vi "Build Param Properties.vi"(0 "Parameter":T1, 5 "error in (no error)":errorcluster) -> (7 "signed":bool, 8 "Prop Names":string[](array[string]), 9 "numberBits":i32, 10 "Prop Values":variant[](array[variant]), 11 "startBit":i32, 13 "scaleFactor":dbl, 16 "name":string, 18 "error out":errorcluster, 19 "scaleOffset":dbl)   [LabVIEW 2013, in "AIT 664 Custom Device.lvlib"]
uses:
  AIT 664 Custom Device.lvlib
  Controls/664 -Param.ctl
  Controls and Global/Global.vi
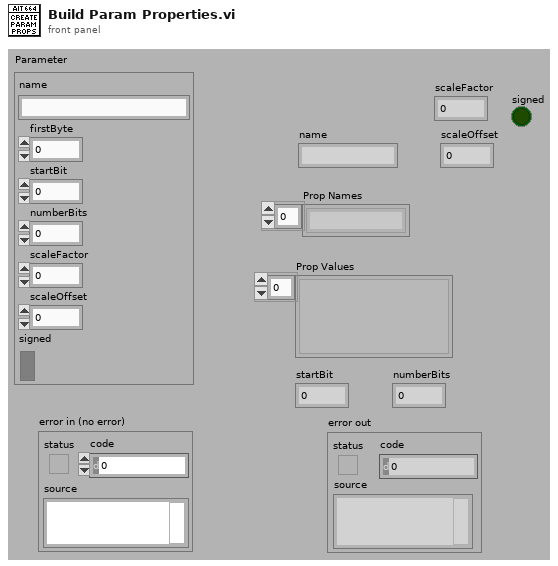
[diagram p1: front panel]
types:
  T1 = typedef "AIT 664 Custom Device.lvlib/664 -Param.ctl" = cluster{"name":string, "firstByte":i32, "startBit":i32, "numberBits":i32, "scaleFactor":dbl, "scaleOffset":dbl, "signed":bool}
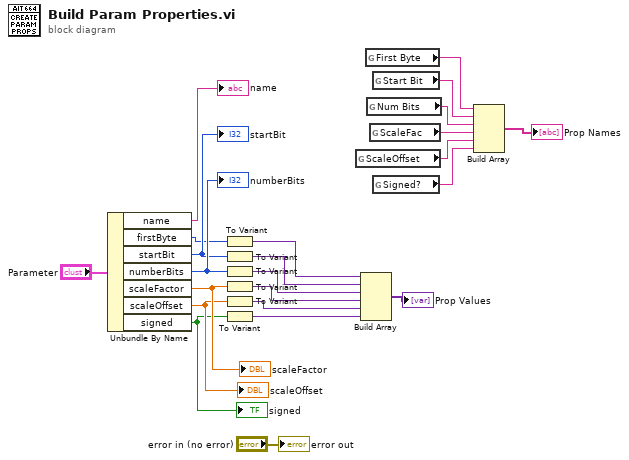
[diagram p0: block diagram]
diagram:
  n1 = Unbundle By Name("Parameter") -> ("name"=→"name":string, "firstByte"=w2:i32, "startBit"=w18:i32, "numberBits"=w22:i32, "scaleFactor"=w12:dbl, "scaleOffset"=w11:dbl, "signed"=w7:bool)
  "startBit" <- w18
  "numberBits" <- w22
  "scaleOffset" <- w11
  "scaleFactor" <- w12
  "signed" <- w7
  n2 = To Variant(anything=w2) -> (Variant=w1:variant)
  n3 = To Variant(anything=w18) -> (Variant=w21:variant)
  n4 = To Variant(anything=w22) -> (Variant=w20:variant)
  n5 = To Variant(anything=w12) -> (Variant=w14:variant)
  n6 = To Variant(anything=w11) -> (Variant=w10:variant)
  n7 = To Variant(anything=w7) -> (Variant=w6:variant)
  n8 = global read "Global.vi" "ScaleOffset"() -> (w9:string)
  n9 = Build Array(w1, w21, w20, w14, w10, w6) -> (→"Prop Values":variant[])
  n10 = global read "Global.vi" "First Byte"() -> (w4:string)
  n11 = global read "Global.vi" "Num Bits"() -> (w17:string)
  n12 = global read "Global.vi" "ScaleFac"() -> (w15:string)
  n13 = global read "Global.vi" "Start Bit"() -> (w16:string)
  n14 = global read "Global.vi" "Signed?"() -> (w8:string)
  n15 = Build Array(w4, w16, w17, w15, w9, w8) -> (→"Prop Names":string[])
  "error out" <- "error in (no error)"
